vi "作业.vi"() -> ()   [LabVIEW 2018]
uses:
  <resource>/objmgr/nicontrollersysapi.rc
  <resource>/objmgr/nisysapi.rc
panel:
  out "System Inf":T1
  out "硬件负载":T2 {"硬盘负载" format="%#.1g%"; "内存负载" format="%#.1g%"; "CPU负荷" format="%#_6g%"; "CPU各核心负载" format="%.0f%"}
  in  "白圆的半径":dbl=5.0
  in  "红圆的半径":dbl=3.0
  out "XY图 2":cluster{dbl[], dbl[]}[](graph)
  out "XY图":cluster{dbl[], dbl[]}(graph)
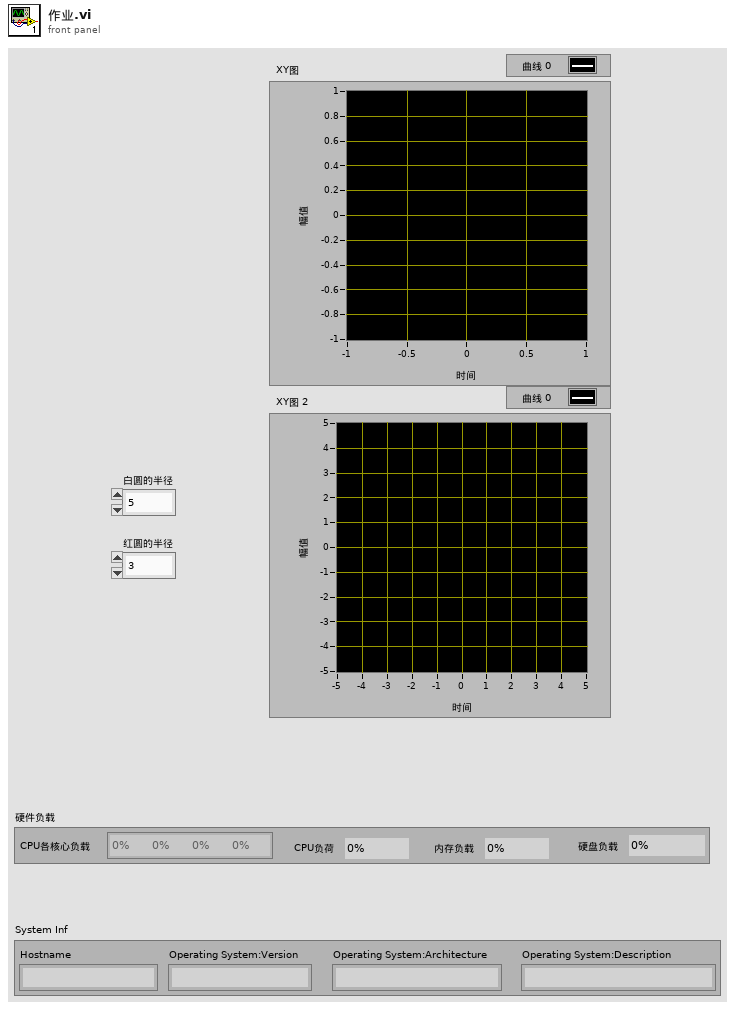
[diagram p1: front panel]
types:
  T1 = cluster{"Hostname":string, "Operating System:Version":string, "Operating System:Architecture":string, "Operating System:Description":string}
  T2 = cluster{"CPU各核心负载":u32[], "CPU负荷":dbl, "内存负载":dbl, "硬盘负载":dbl}
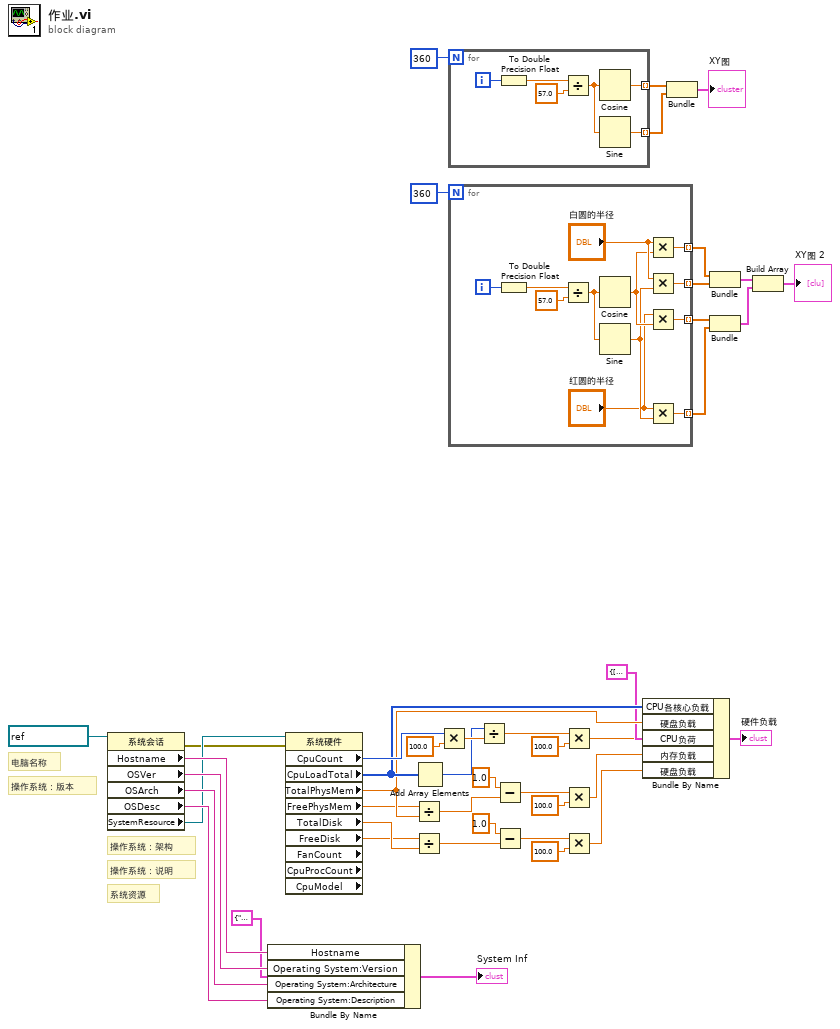
[diagram p0: block diagram]
diagram:
  # "系统资源"
  # "操作系统：说明"
  # "操作系统：架构"
  # "操作系统：版本"
  # "电脑名称"
  n1 = property class="系统会话"(reference=refnum<k21> "localhost" ("Target (localhost)")) -> (error out=w3:errorcluster, "Hostname"=w6:string, "OSVer"=w7:string, "OSArch"=w8:string, "OSDesc"=w9:string, "SystemResource"=w4:refnum<k20>)  [unwired: 1 in, 1 out]
  n2 = Bundle By Name(cluster=T1 {"Hostname"="PC-201906191007", "Operating System:Version"="10.0.17763", "Operating System:Architecture"="Windows x64", "Operating System:Description"="Microsoft Windows 10 专业版"} ("System Inf"), "Hostname"=w6, "Operating System:Version"=w7, "Operating System:Architecture"=w8, "Operating System:Description"=w9) -> (→"System Inf":T1)
  n3 = property class="系统硬件" props=["CpuCount", "CpuLoadTotal", "TotalPhysMem", "FreePhysMem", "TotalDisk", "FreeDisk", "FanCount", "CpuProcCount", "CpuModel"](reference=w4, error in=w3) -> ("CpuCount"=w20:i32, "CpuLoadTotal"=w19:u32[], "TotalPhysMem"=w18:dbl, "FreePhysMem"=w17:dbl, "TotalDisk"=w16:dbl, "FreeDisk"=w15:dbl)  [unwired: 5 out]
  n4 = Divide(x=w17, y=w18) -> (x/y=w28:dbl)
  n5 = Divide(x=w15, y=w16) -> (x/y=w21:dbl)
  n6 = Add Array Elements(numeric array=w19) -> (sum=w31:u32)
  n7 = Multiply(x=w20, y=100.0) -> (x*y=w32:dbl)
  n8 = for {
    N: 360 -> [_]
    tunnel: [w48] -> w44 mode=indexing
    tunnel: [w46] -> w42 mode=indexing
    i -> [w49]
    n9 = To Double Precision Float(number=w49) -> (double precision float=w50:dbl)
    n10 = Divide(x=w50, y=57.0) -> (x/y=w47:dbl)
    n11 = Cosine(x=w47) -> (cos(x)=w46:dbl)
    n12 = Sine(x=w47) -> (sin(x)=w48:dbl)
  }
  n13 = for {
    N: 360 -> [_]
    tunnel: [w57] -> w40 mode=indexing
    tunnel: [w59] -> w39 mode=indexing
    tunnel: [w53] -> w36 mode=indexing
    tunnel: [w52] -> w35 mode=indexing
    i -> [w61]
    n14 = To Double Precision Float(number=w61) -> (double precision float=w62:dbl)
    n15 = Divide(x=w62, y=57.0) -> (x/y=w60:dbl)
    n16 = Cosine(x=w60) -> (cos(x)=w56:dbl)
    n17 = Sine(x=w60) -> (sin(x)=w55:dbl)
    n18 = Multiply(x="白圆的半径", y=w56) -> (x*y=w59:dbl)
    n19 = Multiply(x="白圆的半径", y=w55) -> (x*y=w57:dbl)
    n20 = Multiply(x="红圆的半径", y=w56) -> (x*y=w53:dbl)
    n21 = Multiply(x="红圆的半径", y=w55) -> (x*y=w52:dbl)
  }
  n22 = Divide(x=w31, y=w32) -> (x/y=w30:dbl)
  n23 = Subtract(x=1.0, y=w28) -> (x-y=w25:dbl)
  n24 = Subtract(x=1.0, y=w21) -> (x-y=w24:dbl)
  n25 = Multiply(x=w30, y=100.0) -> (x*y=w13:dbl)
  n26 = Multiply(x=w25, y=100.0) -> (x*y=w12:dbl)
  n27 = Multiply(x=w24, y=100.0) -> (x*y=w11:dbl)
  n28 = Bundle By Name(cluster=T2 {"CPU各核心负载"=[9, 25, 21, 12], "CPU负荷"=16.75, "内存负载"=56.48655429645182, "硬盘负载"=40.29586920045074} ("硬件负载"), "CPU各核心负载"=w19, "硬盘负载"=w18, "CPU负荷"=w13, "内存负载"=w12, "硬盘负载"=w11) -> (→"硬件负载":T2)
  n29 = Bundle(w42, w44) -> (→"XY图":cluster{dbl[], dbl[]})  [unwired: 1 in]
  n30 = Bundle(w39, w40) -> (w38:cluster{dbl[], dbl[]})  [unwired: 1 in]
  n31 = Bundle(w36, w35) -> (w34:cluster{dbl[], dbl[]})  [unwired: 1 in]
  n32 = Build Array(w38, w34) -> (→"XY图 2":cluster{dbl[], dbl[]}[])
